vi "FuseTargeting.vi"(4 "Robot_H (deg)":dbl, 6 "LimeLight Valid":bool, 8 "LimeLight Raw Horizontal Offset (deg)":dbl, 9 "LIDAR Range (in)":dbl, 10 "Estimated Heading to Target (deg)":dbl, 11 "Estimated Distance to Target (in)":dbl) -> (1 "Pointed at Target":bool, 2 "Fused Heading to Target Delta (deg)":dbl, 3 "Fused Distance to Target (in)":dbl)   [LabVIEW 2019]
doc: "This VI fuses data from multiple sensing modalities to estimate the robot's range and heading-error to the target."
uses:
  dsdata.vi
panel:
  in  "Relative LIDAR Weighting":dbl=6.0 format="%#_13g"
  in  "Largest distance disagreement (in)":dbl=100.0 format="%#_13g"
  in  "Loops to Average LIDAR":i32=15
  in  "Min Timed Aligned (ms)":u32=200
  in  "Acceptable Heading Error (deg)":dbl=5.0
  in  "Loops to Average LL":i32=15
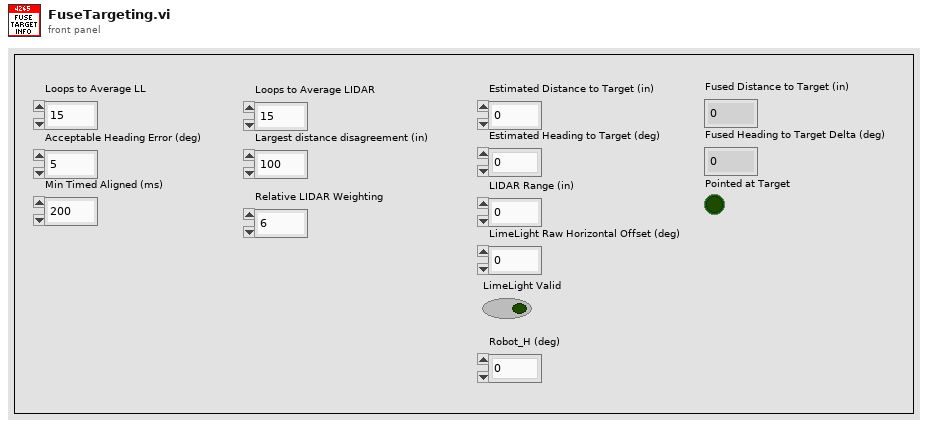
[diagram p1: front panel]
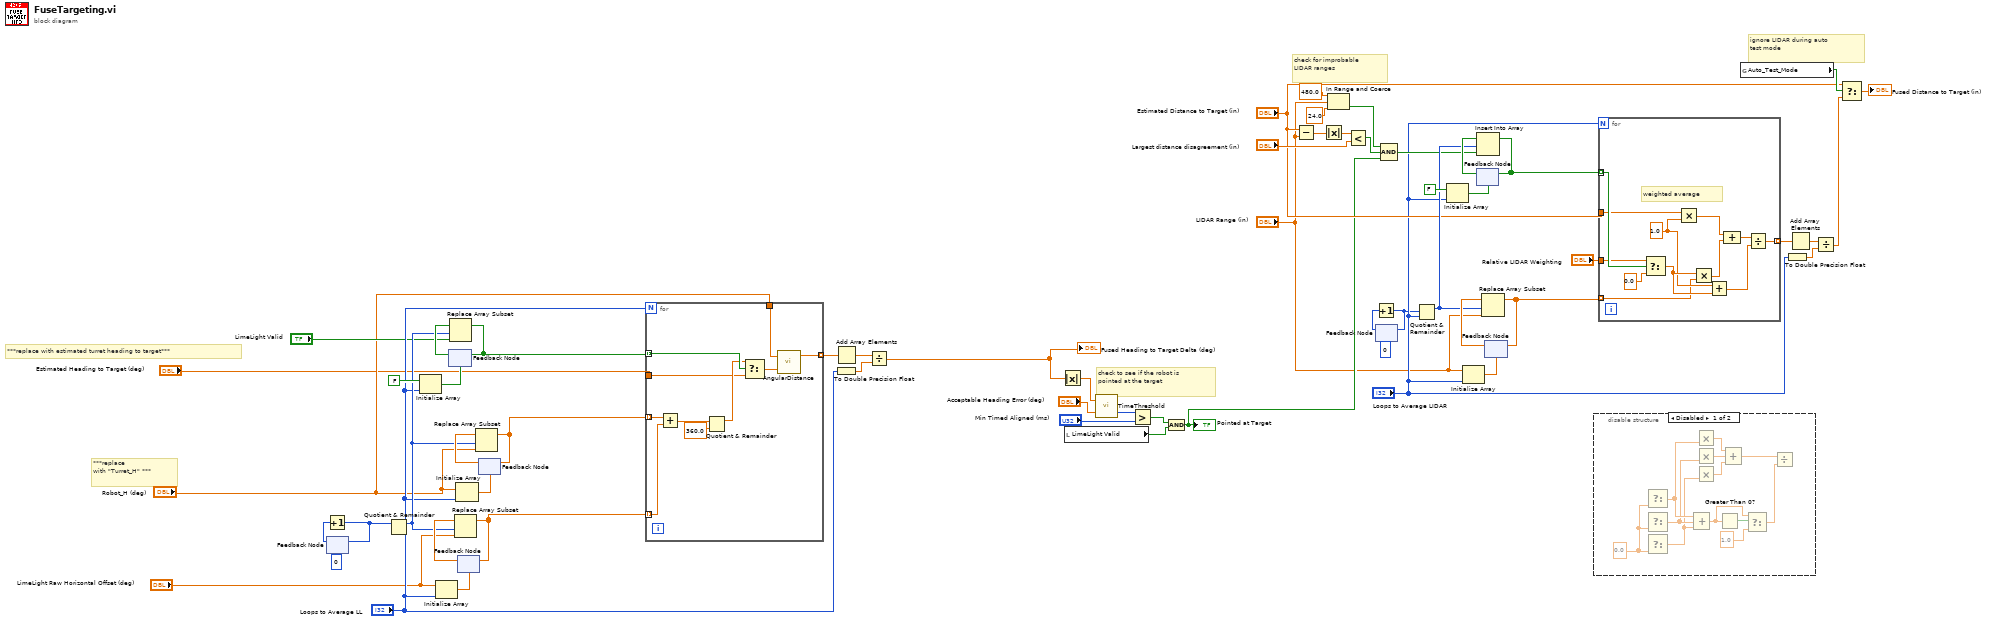
[diagram p0: block diagram]
diagram:
  # "check for improbable\nLIDAR ranges"
  # "check to see if the robot is\npointed at the target"
  # "ignore LIDAR during auto\ntest mode"
  # "***replace \nwith \"Turret_H\" ***"
  # "***replace with estimated turret heading to target***"
  n1 = feedback #1(0) -> (w56:i32)
  n2 = Increment(x=w56) -> (x+1=w55:i32)
  n3 = feedback-in #1(w55) -> ()
  n4 = Quotient & Remainder(x=w55, y="Loops to Average LL") -> (x-y*floor(x/y)=w47:i32)  [unwired: 1 out]
  n5 = Initialize Array(FALSE, "Loops to Average LL") -> (w52:bool[])
  n6 = Initialize Array("LimeLight Raw Horizontal Offset (deg)", "Loops to Average LL") -> (w59:dbl[])
  n7 = feedback #2(w52) -> (w54:bool[])
  n8 = Replace Array Subset(array=w54, new element="LimeLight Valid", index=w47) -> (w51:bool[])
  n9 = feedback-in #2(w51) -> ()
  n10 = Initialize Array("Robot_H (deg)", "Loops to Average LL") -> (w49:dbl[])
  n11 = feedback #3(w59) -> (w58:dbl[])
  n12 = Replace Array Subset(array=w58, new element="LimeLight Raw Horizontal Offset (deg)", index=w47) -> (w50:dbl[])
  n13 = feedback-in #3(w50) -> ()
  n14 = feedback #4(w49) -> (w48:dbl[])
  n15 = Replace Array Subset(array=w48, new element="Robot_H (deg)", index=w47) -> (w46:dbl[])
  n16 = feedback-in #4(w46) -> ()
  n17 = for {
    N: "Loops to Average LL" -> [_]
    tunnel: w51 -> [w69] mode=indexing
    tunnel: w50 -> [w66] mode=indexing
    tunnel: "Estimated Heading to Target (deg)" -> [w64]
    tunnel: w46 -> [w63] mode=indexing
    tunnel: "Robot_H (deg)" -> [w62]
    tunnel: [w60] -> w45 mode=indexing
    n18 = Add(x=w63, y=w66) -> (x+y=w68:dbl)
    n19 = Quotient & Remainder(x=w68, y=360.0) -> (x-y*floor(x/y)=w65:dbl)  [unwired: 1 out]
    n20 = Select(t=w65, s=w69, f=w64) -> (s? t:f=w61:dbl)
    n21 = call "AngularDistance.vi"("Goal Angle (deg) [0,360]"=w61, "Current Angle (deg) [-Inf,+Inf]"=w62) -> ("Signed Angular Distance (deg) [-180,+180]"=w60:dbl)  [unwired: 1 out]
  }
  n22 = Add Array Elements(numeric array=w45) -> (sum=w44:dbl)
  n23 = To Double Precision Float(number="Loops to Average LL") -> (double precision float=w43:dbl)
  n24 = Divide(x=w44, y=w43) -> (x/y=w1:dbl)
  "Fused Heading to Target Delta (deg)" <- w1
  n25 = Absolute Value(x=w1) -> (abs(x)=w36:dbl)
  n26 = local read "LimeLight Valid"() -> (w31:bool)
  n27 = call "TimeThreshold.vi"("Threshold"="Acceptable Heading Error (deg)", "Current Value"=w36) -> ("Time Below Threshold (ms)"=w34:u32)  [unwired: 1 out]
  n28 = Greater?(x=w34, y="Min Timed Aligned (ms)") -> (0:w32:bool)
  n29 = Compound Arithmetic op=AND(w32, w31) -> (w10:bool)
  "Pointed at Target" <- w10
  n30 = Subtract(x="Estimated Distance to Target (in)", y="LIDAR Range (in)") -> (x-y=w30:dbl)
  n31 = Absolute Value(x=w30) -> (abs(x)=w29:dbl)
  n32 = In Range and Coerce(upper limit=480.0, x="LIDAR Range (in)", lower limit=24.0) -> (In Range?=w5:bool)  [unwired: 1 out]
  n33 = Less?(x=w29, y="Largest distance disagreement (in)") -> (x < y?=w27:bool)
  n34 = feedback #5(0) -> (w8:i32)
  n35 = Increment(x=w8) -> (x+1=w7:i32)
  n36 = feedback-in #5(w7) -> ()
  n37 = Compound Arithmetic op=AND(w5, w27, w10) -> (w15:bool)
  n38 = Quotient & Remainder(x=w7, y="Loops to Average LIDAR") -> (x-y*floor(x/y)=w19:i32)  [unwired: 1 out]
  n39 = Initialize Array(FALSE, "Loops to Average LIDAR") -> (w22:bool[])
  n40 = Initialize Array("LIDAR Range (in)", "Loops to Average LIDAR") -> (w26:dbl[])
  n41 = feedback #6(w22) -> (w24:bool[])
  n42 = Insert Into Array(array=w24, index=w19, new element=w15) -> (w21:bool[])
  n43 = feedback-in #6(w21) -> ()
  n44 = feedback #7(w26) -> (w25:dbl[])
  n45 = Replace Array Subset(array=w25, new element="LIDAR Range (in)", index=w19) -> (w20:dbl[])
  n46 = feedback-in #7(w20) -> ()
  n47 = disable-structure shown="Disabled" {
    frame Disabled {
      w74 = 0.0 ("f")
      n48 = Select(f=w74) -> (s? t:f=w78:dbl)  [unwired: 2 in]
      n49 = Select(f=w74) -> (s? t:f=w77:dbl)  [unwired: 2 in]
      n50 = Select(f=w74) -> (s? t:f=w76:dbl)  [unwired: 2 in]
      n51 = Compound Arithmetic op=unknown(w78, w77, w76) -> (w72:dbl)
      n52 = Multiply(y=w78) -> (x*y=w80:dbl)  [unwired: 1 in]
      n53 = Multiply(y=w77) -> (x*y=w79:dbl)  [unwired: 1 in]
      n54 = Multiply(y=w76) -> (x*y=w75:dbl)  [unwired: 1 in]
      n55 = Greater Than 0?(x=w72) -> (x > 0?=w73:bool)
      n56 = Compound Arithmetic op=ADD(w80, w79, w75) -> (w81:dbl)
      n57 = Select(t=w72, s=w73, f=1.0) -> (s? t:f=w71:dbl)
      n58 = Divide(x=w81, y=w71) -> ()  [unwired: 1 out]
    }
    frame Enabled {
    }
  }
  n59 = for {
    N: "Loops to Average LIDAR" -> [_]
    tunnel: w21 -> [w86] mode=indexing
    tunnel: w20 -> [w85] mode=indexing
    tunnel: "Estimated Distance to Target (in)" -> [w84]
    tunnel: [w83] -> w18 mode=indexing
    tunnel: "Relative LIDAR Weighting" -> [w82]
    w87 = 1.0 ("x")
    # "weighted average"
    n60 = Select(t=w82, s=w86, f=0.0) -> (s? t:f=w93:dbl)
    n61 = Multiply(x=w84, y=w87) -> (x*y=w90:dbl)
    n62 = Multiply(x=w93, y=w85) -> (x*y=w91:dbl)
    n63 = Add(x=w87, y=w93) -> (x+y=w92:dbl)
    n64 = Compound Arithmetic op=ADD(w90, w91) -> (w89:dbl)
    n65 = Divide(x=w89, y=w92) -> (x/y=w83:dbl)
  }
  n66 = global read "dsdata.vi" "Auto_Test_Mode"() -> (w37:bool)
  n67 = To Double Precision Float(number="Loops to Average LIDAR") -> (double precision float=w16:dbl)
  n68 = Add Array Elements(numeric array=w18) -> (sum=w17:dbl)
  n69 = Divide(x=w17, y=w16) -> (x/y=w12:dbl)
  n70 = Select(t="Estimated Distance to Target (in)", s=w37, f=w12) -> (s? t:f=→"Fused Distance to Target (in)":dbl)
